vi "flash_write_test.vi"   [LabVIEW 2022 SP3]
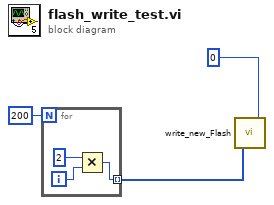
[diagram p0: block diagram]
diagram:
  n1 = for {
    N: 200 -> [_]
    tunnel: [w5] -> w1 mode=indexing
    i -> [w6]
    n2 = Multiply(x=2, y=w6) -> (x*y=w5:i32)
  }
  n3 = call "write_new_Flash.vi"("address (3 bytes)"=u32 0, "write array"=w1) -> ()
